vi "Common-DateTimeToU16Array.vi"(11 "时间标识":timestamp) -> (3 "U16Array":u16[](array[numeric]))   [LabVIEW 2014]
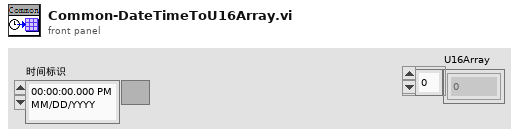
[diagram p1: front panel]
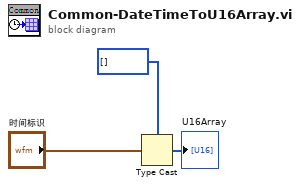
[diagram p0: block diagram]
diagram:
  n1 = Type Cast(type=u16[] [], x="时间标识") -> (*(type *) &x=→"U16Array":u16[])
